vi "3.vi"() -> ()   [LabVIEW 2015]
panel:
  out "最大值":dbl
  out "最小值":dbl
  out "平均值":dbl
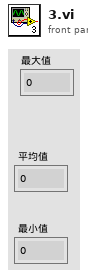
[diagram p1: front panel]
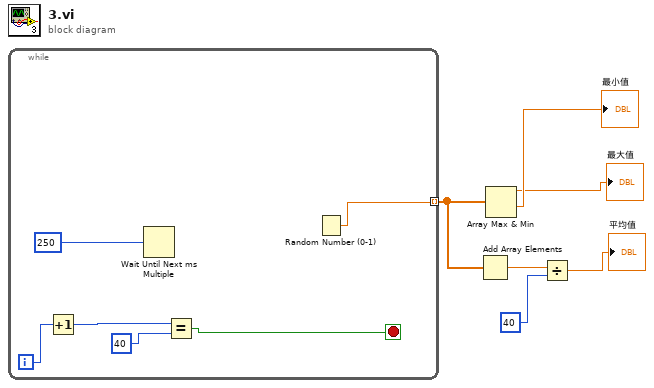
[diagram p0: block diagram]
diagram:
  n1 = while {
    tunnel: [w7] -> w1 mode=indexing
    i -> [w9]
    stop <- w8 stop-if-true
    n2 = Increment(x=w9) -> (x+1=w10:i32)
    n3 = Wait Until Next ms Multiple(millisecond multiple=250) -> ()  [unwired: 1 out]
    n4 = Equal?(x=w10, y=40) -> (x = y?=w8:bool)
    n5 = Random Number (0-1)() -> (number: 0 to 1=w7:dbl)
  }
  n6 = Add Array Elements(numeric array=w1) -> (sum=w6:dbl)
  n7 = Array Max & Min(array=w1) -> (max value=→"最大值":dbl, min value=→"最小值":dbl)  [unwired: 2 out]
  n8 = Divide(x=w6, y=40) -> (x/y=→"平均值":dbl)
